vi "23384_Davis_Poku_Amankwa_Amankwa.DavisPoku.MNE1201.2.DIY_348253_1771596509.vi"() -> ()   [LabVIEW 2018]
panel:
  in  "stop":bool
  out "Elapsed Time(second)":dbl
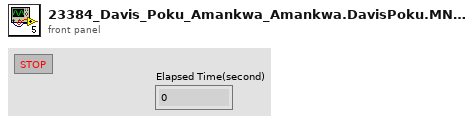
[diagram p1: front panel]
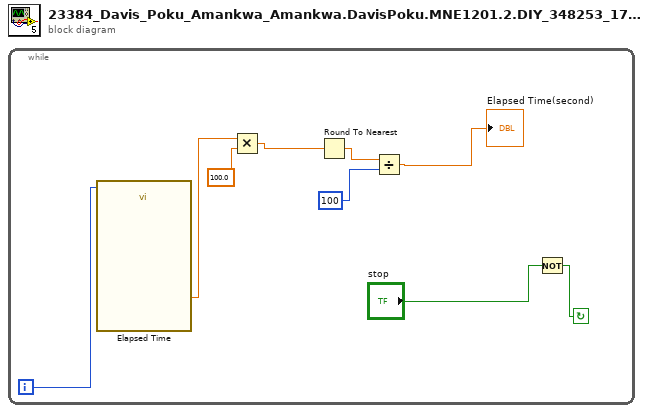
[diagram p0: block diagram]
diagram:
  n1 = while {
    i -> [w1]
    stop <- w8 continue-if-true
    n2 = call "Elapsed Time"("Time Target (s)"=w1) -> ("Elapsed Time (s)"=w5:dbl)  [unwired: 11 in, 7 out]
    n3 = Multiply(x=w5, y=100.0) -> (x*y=w3:dbl)
    n4 = Round To Nearest(number=w3) -> (nearest integer value=w2:dbl)
    n5 = Divide(x=w2, y=100) -> (x/y=→"Elapsed Time(second)":dbl)
    n6 = Not(x="stop") -> (.not. x?=w8:bool)
  }
